vi "Test Data Path.vi"() -> (3 "Test Data Path":path)   [LabVIEW 2020]
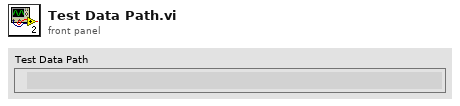
[diagram p1: front panel]
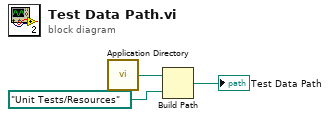
[diagram p0: block diagram]
diagram:
  n1 = call <vilib>:"Application Directory.vi"() -> ("Application Directory"=w2:path)
  n2 = Build Path(base path=w2, name or relative path=path "Unit Tests/Resources") -> (appended path=→"Test Data Path":path)
